vi "Co-ordinate Prediction.vi"(8 "theta (deg)":dbl format="%#_13g", 10 "Y Top":dbl format="%#_13g", 11 "X Top":dbl format="%#_8g") -> (2 "Y Pred":dbl, 3 "X Pred":dbl format="%.6g")   [LabVIEW 2018]
panel:
  out "Y out":dbl
  out "X out":dbl format="%#_13g"
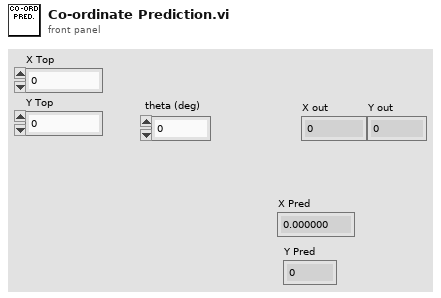
[diagram p1: front panel]
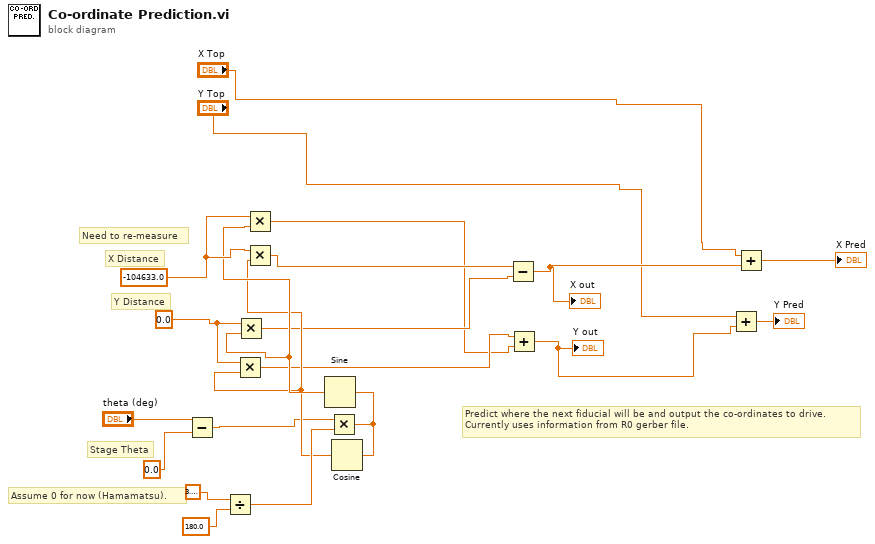
[diagram p0: block diagram]
diagram:
  w15 = 0.0 ("Y dist")
  w16 = -104633.0 ("X dist")
  # "Assume 0 for now (Hamamatsu)."
  # "Need to re-measure"
  # "Stage Theta"
  # "Y Distance"
  # "X Distance"
  # "Predict where the next fiducial will be and output the co-ordinates to drive.\nCurrently uses information from R0 gerber file."
  n1 = Subtract(x="theta (deg)", y=0.0) -> (x-y=w1:dbl)
  n2 = Divide(x=3.141592653589793, y=180.0) -> (x/y=w19:dbl)
  n3 = Multiply(x=w1, y=w19) -> (x*y=w17:dbl)
  n4 = Sine(x=w17) -> (sin(x)=w14:dbl)
  n5 = Multiply(x=w15, y=w14) -> (x*y=w11:dbl)
  n6 = Multiply(x=w16, y=w14) -> (x*y=w9:dbl)
  n7 = Cosine(x=w17) -> (cos(x)=w13:dbl)
  n8 = Multiply(x=w15, y=w13) -> (x*y=w10:dbl)
  n9 = Multiply(x=w16, y=w13) -> (x*y=w12:dbl)
  n10 = Subtract(x=w12, y=w11) -> (x-y=w8:dbl)
  "X out" <- w8
  n11 = Add(x=w10, y=w9) -> (x+y=w7:dbl)
  "Y out" <- w7
  n12 = Add(x="Y Top", y=w7) -> (x+y=→"Y Pred":dbl)
  n13 = Add(x="X Top", y=w8) -> (x+y=→"X Pred":dbl)
